vi "QBacklight.vi"(8 "error in (no error)":errorcluster, 11 "VISA resource name":refnum<visa-resource-name>) -> (0 "error out":errorcluster, 2 "BKLT State":u32(ring) items=["Off", "Low", "High"], 3 "VISA resource name out":refnum<visa-resource-name>)   [LabVIEW 2009, in "Newport 1830-C.lvlib"]
doc: "0=off\n1=low\n2=high"
uses:
  Newport 1830-C.lvlib
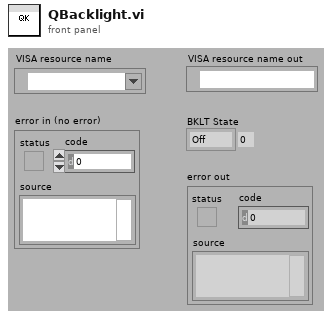
[diagram p1: front panel]
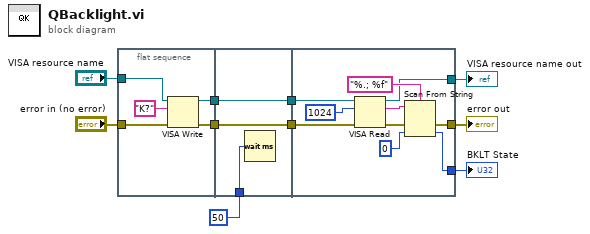
[diagram p0: block diagram]
diagram:
  n1 = flat-sequence {
    tunnel: [w14] -> w10
    tunnel: [w13] -> w9
    tunnel: "error in (no error)" -> [w12]
    tunnel: "VISA resource name" -> [w11]
    tunnel: [w18] -> w8
    tunnel: w10 -> [w18]
    tunnel: w9 -> [w17]
    tunnel: [w17] -> w7
    tunnel: u32 50 ("Delay Time (s)") -> [w16]
    tunnel: [w23] -> w4
    tunnel: [w22] -> w3
    tunnel: w8 -> [w21]
    tunnel: w7 -> [w20]
    tunnel: [w19] -> w5
    frame #0 {
      n2 = VISA Write(VISA resource name=w11, write buffer="K?" ("command"), error in (no error)=w12) -> (VISA resource name out=w14:refnum<visa-resource-name>, error out=w13:errorcluster)  [unwired: 1 out]
    }
    frame #1 {
      n3 = Wait (ms)(milliseconds to wait=w16) -> ()  [unwired: 1 out]
    }
    frame #2 {
      n4 = VISA Read(VISA resource name=w21, byte count=u32 1024, error in (no error)=w20) -> (VISA resource name out=w23:refnum<visa-resource-name>, read buffer=w25:string, error out=w27:errorcluster)  [unwired: 1 out]
      n5 = Scan From String(format string="%.; %f", input string=w25, error in=w27, default 1=u32 0 ("default value 1")) -> (error out=w22:errorcluster, output 1=w19:u32)  [unwired: 1 in, 2 out]
    }
  }
  "VISA resource name out" <- w4
  "error out" <- w3
  "BKLT State" <- w5
